vi "05-ShiftRegister.vi"() -> ()   [LabVIEW 2014]
panel:
  in  "stop":bool
  out "x-3a":dbl
  out "x-2a":dbl
  out "x-a":dbl
  out "x":dbl
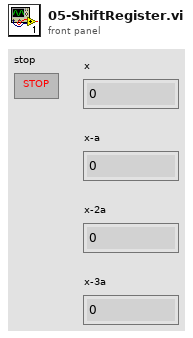
[diagram p1: front panel]
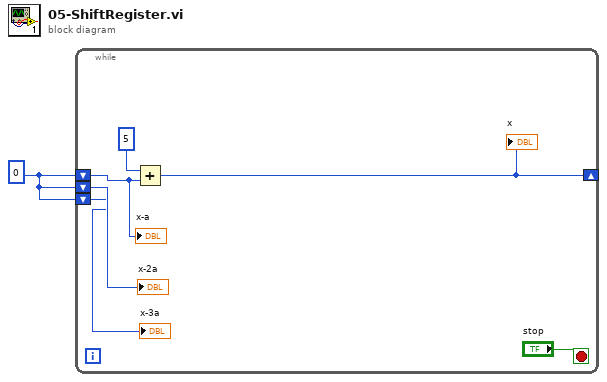
[diagram p0: block diagram]
diagram:
  w1 = 0
  n1 = while {
    shift-right: [w6] -> _
    shift-left: w1 -> [w5]
    shift-left: w1 -> [w3]
    shift-left: w1 -> [w4]
    stop <- "stop" stop-if-true
    n2 = Add(x=5, y=w5) -> (x+y=w6:i32)
    "x" <- w6
    "x-a" <- w5
    "x-2a" <- w4
    "x-3a" <- w3
  }
